vi "PSTR Controller.vi"(11 "Expt State (in)":T6) -> (3 "Expt State":T6)   [LabVIEW 2020]
uses:
  CFTS Main Panel SubVIs/CFTS-Experiment State.ctl
  epl-vi-lib/Utility VIs/Type Defs/Left-Right ring.ctl
  <vilib>/printing/EasyPrintingControls.llb/layout_options.ctl
  <vilib>/printing/EasyPrintingControls.llb/orientation.ctl
  <vilib>/printing/EasyPrintingControls.llb/panel_scaling_for_page.ctl
  <vilib>/printing/EasyPrintingControls.llb/margins.ctl
  <vilib>/printing/EasyPrintingControls.llb/margin_values.ctl
  <vilib>/printing/EasyPrintingControls.llb/measurement_system.ctl
  <vilib>/printing/EasyPrintingControls.llb/printer_options.ctl
  <vilib>/printing/EasyPrintingControls.llb/printing_method.ctl
  <vilib>/printing/EasyPrintingControls.llb/color_or_monochrome.ctl
  <vilib>/printing/EasyPrintingControls.llb/page_header_options.ctl
  <vilib>/printing/EasyPrintingControls.llb/page_headers.ctl
  <vilib>/printing/EasyPrintingControls.llb/page_header_content_options.ctl
  epl-vi-lib/Utility VIs/Buttons/KCheckmarkBoolean 2.ctl
  Typedefs/PSTR-Parameters.ctl
  Typedefs/PSTR-Stimulus Params.ctl
  Typedefs/PSTR-FreqSeq Params.ctl
  Typedefs/PSTR-LevelSeq Params.ctl
  Typedefs/PSTR-SeqParams.ctl
  Typedefs/PSTR-Response Params.ctl
  Typedefs/PSTR-Hidden Params.ctl
  Typedefs/PSTR-Window Shape.ctl
  Typedefs/PSTR-Data.ctl
  Typedefs/PSTR-Model Fit.ctl
  Typedefs/PSTR-Fit Parameters.ctl
  <vilib>/printing/EasyPrintingControls.llb/contents.ctl
  Typedefs/PSTR-Measurement State.ctl
  <vilib>/printing/EasyPrinting.llb/Easy Print VI Panel or Documentation (refnum).vi
  <vilib>/Utility/NIReport.llb/NI_ReportGenerationCore.lvlib
panel:
  in  "LevelSeq":T1={"Min (dB)"=0.0, "Max (dB)"=80.0, "Step (dB)"=20.0}
  in  "FreqSeq":T2={"Min (kHz)"=4.0, "Max (kHz)"=64.0, "Step (oct)"=0.5}
  in  "Seq":T3={"Order"=enum."Sequential", "Averages"=20}
  in  "Response":cluster{"Grass gain":dbl, "Window (ms)":dbl}={"Grass gain"=10000.0, "Window (ms)"=10000.0}
  in  "Stim":T5={"Ear"=enum."Right", "BW (oct)"=0.25, "Seed"=37, "Ramp (ms)"=5.0, "On time (ms)"=300.0, "Off time (ms)"=300.0, "Delay (ms)"=5.0}
  out "User":string
  out "Run #":u16
  out "ID #":u16
  out "Path":path
  out "Result":T7
  in  "Tab":enum32{"Recording", "Gain", "PSTR"}(tab)
  out "reject":bool
  out "Status":string
  out "Waveform":cluster{dbl, "dx":dbl, "Y":dbl[]}[](graph)
  out "Spectrum":cluster{dbl, "dx":dbl, "Y":dbl[]}[](graph)
  in  "RejThr":dbl=30.0 caption="Rej Thresh µV"
  in  "Override":bool
  in  "iFreq":u16(ring) items=["0.75 kHz"]
  out "Gain":cluster{"Array":dbl[], "Array":dbl[]}[](graph)
  in  "Legend":i32(listbox)
  out "vsFreq":cluster{"Array":dbl[], "Array":dbl[]}[](graph)
  in  "Show fits":T8
  in  "iFreq 2":u16(ring) items=["0.75 kHz"]
  in  "Legend 2":i32(listbox)
  out "PSTH":cluster{"Array":dbl[], "Array":dbl[]}[](graph)
  in  "Separation (uV)":dbl
  out "FitSummary":cluster{"Array":dbl[], "Array":dbl[]}[](graph)
  in  "Start":bool
  in  "Stop":bool
  out "Progress":cluster{"freq":i32, "level":i32} {"level" scale=0.0..2.0; "freq" scale=0.0..1.0}
  in  "layout options":T9={"orientation (unchanged)"=0, "panel scaling for page (unchanged)"=0, "margins"={"override VI margins (false)"=FALSE, "margins (1.00)"={"top"=1.0, "left"=1.0, "right"=1.0, "bottom"=1.0}, "measurement system (default)"=0}, "printer options"={"destination printer name (current)"="", "printing method (unchanged)"=0, "color or monochrome (unchanged)"=0}, "page header options"={"page headers (unchanged)"=0, "page header content options"={"Include VI Name"=TRUE, "Include VI Path"=TRUE, "Include Last Modification Date"=TRUE, "Include Date Printed"=TRUE, "Include Page Number"=TRUE, "Include VI Icon"=TRUE}}} {"page header options"."page headers (unchanged)" items=["Unchanged", "Include page headers", "Do not include page headers"]; "printer options"."color or monochrome (unchanged)" items=["Unchanged", "Color/grayscale", "Monochrome"]; "printer options"."printing method (unchanged)" items=["Unchanged", "Standard", "PostScript", "Bitmap"]; "panel scaling for page (unchanged)" items=["Unchanged", "No Scaling", "Scale front panel to fit"]; "orientation (unchanged)" items=["Unchanged", "portrait", "landscape"]; "margins"."measurement system (default)" items=["Default", "US", "Metric"]; "margins"."margins (1.00)"."right" format="%.2f"; "margins"."margins (1.00)"."bottom" format="%.2f"; "margins"."margins (1.00)"."top" format="%.2f"; "margins"."margins (1.00)"."left" format="%.2f"}
  in  "RETURN":bool
  # "Stimulus"
  # "Frequency"
  # "Level"
  # "Sequence"
  # "Response"
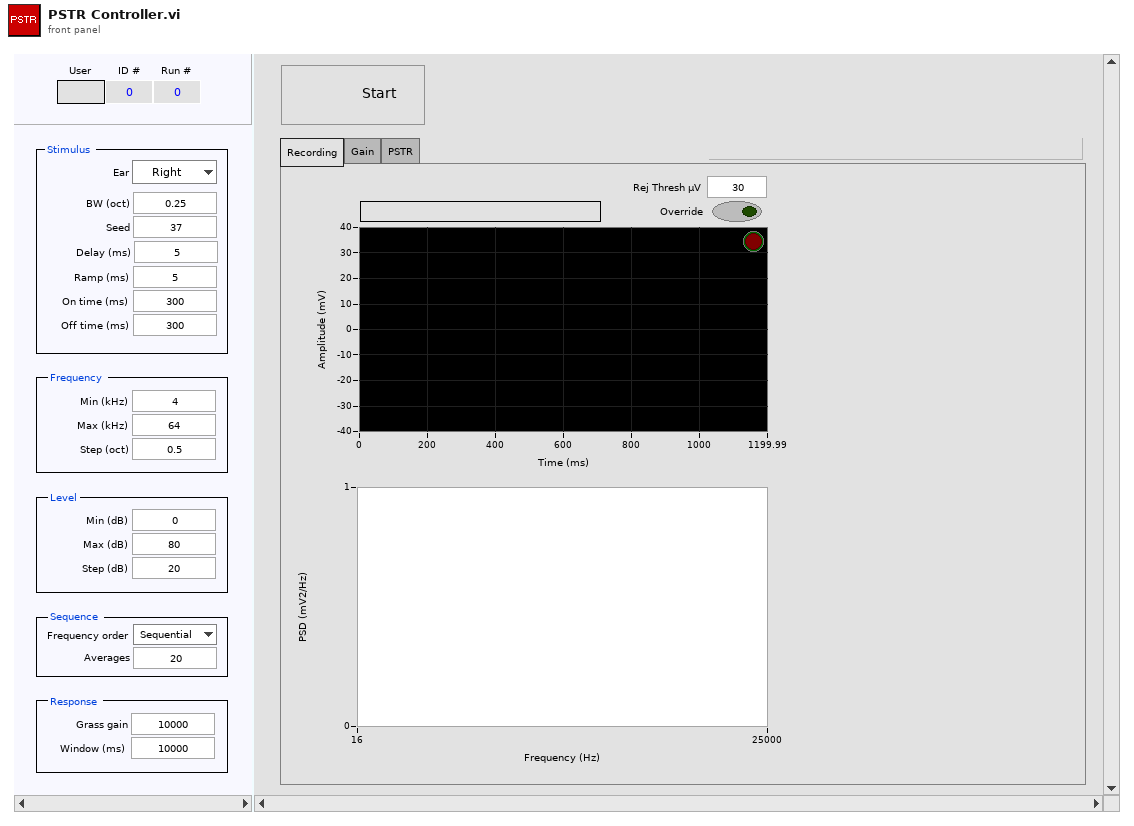
[diagram p1: front panel]
types:
  T1 = cluster{"Min (dB)":dbl, "Max (dB)":dbl, "Step (dB)":dbl}
  T2 = cluster{"Min (kHz)":dbl, "Max (kHz)":dbl, "Step (oct)":dbl}
  T3 = cluster{"Order":enum16{"Sequential", "Random"}, "Averages":i32}
  T4 = typedef "Left-Right ring.ctl" = enum16{"Right", "Left"}
  T5 = cluster{"Ear":T4, "BW (oct)":dbl, "Seed":i32, "Ramp (ms)":dbl, "On time (ms)":dbl, "Off time (ms)":dbl, "Delay (ms)":dbl}
  T6 = typedef "CFTS-Experiment State.ctl" = cluster{"Experimenter":string, "Number":u32, "Right":string, "Left":string, "Data Folder":path, "State File":path, "Version Info":string, "End Exposure Time":dbl, "Exposure Duration":string, "Run #":cluster{"CAP":i16, "ABR":i16, "DP":i16, "VsEP":i16, "MeasSeq":i16, "SubSeq":i16, "SFOAE":i16}}
  T7 = cluster{"iLevel":i32, "done":bool, "abort":bool, "PSD":dbl[][], "error":errorcluster, "spont":bool, "PSTH":dbl[]}
  T8 = typedef "KCheckmarkBoolean 2.ctl" = bool
  T9 = typedef "NI_ReportGenerationCore.lvlib/layout_options.ctl" = cluster{"orientation (unchanged)":T10, "panel scaling for page (unchanged)":T11, "margins":T12, "printer options":T15, "page header options":T18}
  T10 = typedef "NI_ReportGenerationCore.lvlib/orientation.ctl" = u16
  T11 = typedef "NI_ReportGenerationCore.lvlib/panel_scaling_for_page.ctl" = u16
  T12 = typedef "NI_ReportGenerationCore.lvlib/margins.ctl" = cluster{"override VI margins (false)":bool, "margins (1.00)":T13, "measurement system (default)":T14}
  T13 = typedef "NI_ReportGenerationCore.lvlib/margin_values.ctl" = cluster{"top":dbl, "left":dbl, "right":dbl, "bottom":dbl}
  T14 = typedef "NI_ReportGenerationCore.lvlib/measurement_system.ctl" = u16
  T15 = typedef "NI_ReportGenerationCore.lvlib/printer_options.ctl" = cluster{"destination printer name (current)":string, "printing method (unchanged)":T16, "color or monochrome (unchanged)":T17}
  T16 = typedef "NI_ReportGenerationCore.lvlib/printing_method.ctl" = u16
  T17 = typedef "NI_ReportGenerationCore.lvlib/color_or_monochrome.ctl" = u16
  T18 = typedef "NI_ReportGenerationCore.lvlib/page_header_options.ctl" = cluster{"page headers (unchanged)":T19, "page header content options":T20}
  T19 = typedef "NI_ReportGenerationCore.lvlib/page_headers.ctl" = u16
  T20 = typedef "NI_ReportGenerationCore.lvlib/page_header_content_options.ctl" = cluster{"Include VI Name":bool, "Include VI Path":bool, "Include Last Modification Date":bool, "Include Date Printed":bool, "Include Page Number":bool, "Include VI Icon":bool}
  T21 = typedef "PSTR-Data.ctl" = cluster{"Freq":dbl[], "Level":dbl[], "order":i32[], "PSD":dbl[][][][], "Gain":dbl[][][], "Index":dbl[][], "iFreq":i32, "df":dbl, "User":string, "ID":i32, "Run":i32, "iLevel":i32, "finished":bool, "resumed":bool, "Spont":dbl[][], "PSTR":dbl[][][], "dt":dbl, "delay":dbl, "durat":dbl, "Fits":T22[][], "Amplitude":dbl[][]}
  T22 = typedef "PSTR-Model Fit.ctl" = cluster{"Parameters":T23, "t":dbl[], "y":dbl[], "R2":dbl}
  T23 = typedef "PSTR-Fit Parameters.ctl" = cluster{"Ar":dbl, "Tr":dbl, "Ast":dbl, "Tst":dbl, "Ass":dbl}
  T24 = typedef "PSTR-Parameters.ctl" = cluster{"Stimulus":T25, "FreqSeq":T26, "LevelSeq":T27, "Seq":T28, "Response":T29, "Hidden":T30, "RejThr":dbl}
  T25 = typedef "PSTR-Stimulus Params.ctl" = cluster{"Ear":T4, "BW (oct)":dbl, "Seed":i32, "Ramp (ms)":dbl, "On time (ms)":dbl, "Off time (ms)":dbl, "Delay (ms)":dbl}
  T26 = typedef "PSTR-FreqSeq Params.ctl" = cluster{"Min (kHz)":dbl, "Max (kHz)":dbl, "Step (oct)":dbl}
  T27 = typedef "PSTR-LevelSeq Params.ctl" = cluster{"Min (dB)":dbl, "Max (dB)":dbl, "Step (dB)":dbl}
  T28 = typedef "PSTR-SeqParams.ctl" = cluster{"Order":enum16{"Sequential", "Random"}, "Averages":i32}
  T29 = typedef "PSTR-Response Params.ctl" = cluster{"Grass gain":dbl, "Window (ms)":dbl}
  T30 = typedef "PSTR-Hidden Params.ctl" = cluster{"Sample rate (Hz)":dbl, "Nfft":i32, "save raw":bool, "sep":dbl, "Window":T31}
  T31 = typedef "PSTR-Window Shape.ctl" = enum16{"NONE", "Hamming"}
  T32 = enum8{"Enabled", "Disabled", "Disabled and Grayed Out"}
  T33 = typedef "NI_ReportGenerationCore.lvlib/contents.ctl" = u16
  T34 = cluster{"PSTR Params":T24, "Freq":dbl, i32, "Run":i32}
  T35 = cluster{"PSTR Params":T24, "Freq":dbl, "iLevel":i32, "Run":i32}
  T36 = typedef "PSTR-Measurement State.ctl" = enum16{"Init", "Next", "Measure", "End"}
  T37 = enum16{"open", "replace", "create", "open or create", "replace or create", "replace or create with confirmation"}
  T38 = typedef "PSTR-Runtime Data.ctl" = cluster{"Fs":dbl, "AOpts":i32, "stimChan":T39, "len":i32, "offset1":i32, "iLevel":i32, "AOChan":i32[], "Level":dbl[], "nacc":i32, "nrej":i32, "nacq":i32, "abort":bool, "offset2":i32, "gain":dbl, "Nfft":i32, "Neural":dbl[], "Micro":dbl[], "raw":refnum<file>, "spont":bool, "PSTR":dbl[], "trialLen":i32, "gate":dbl[], "window":u16, "BP":cluster{"reverse":dbl[], "forward":dbl[]}, "Smooth":cluster{"reverse":dbl[], "forward":dbl[]}}
  T39 = typedef "Stimulus Channel (Full).xctl/Full Stimulus Channel Data.ctl" = cluster{"Waveform":T40, "Filter":T57, "Burst":T59, "Level":T60, "Name":string, "Advanced":T62, "SAM":T63}
  T40 = typedef "Waveform XCtl.xctl/Waveform Data.ctl" = cluster{"Type":T41, "Tone":T42, "Pulse Train":T43, "Noise":T46, "File":T47, "FMSweep":T48, "Chirp Train":T49, "Complex Tone":cluster{"Params":T51, "Data":T53}, "Moving Ripple":T54}
  T41 = typedef "Waveform Enum.ctl" = enum16{"OFF", "Tone", "Noise", "Pulse Train", "File", "FM Sweep", "Chirp Train", "Complex Tone", "FM Tone", "Moving Ripple"}
  T42 = typedef "Tone Params.ctl" = cluster{"Frequency (kHz)":dbl, "Last Freq":dbl, "Last Phase":dbl}
  T43 = typedef "Pulse Train Params.ctl" = cluster{"Pulse width (us)":dbl, "Pulse rate (Hz)":dbl, "Gap (ms)":dbl, "Polarity":T44, "PT State":T45, "Asynch":bool}
  T44 = typedef "Pulse Polarity.ctl" = enum16{"POS", "NEG", "POS-NEG", "NEG-POS"}
  T45 = typedef "PT-Continuous State.ctl" = cluster{"Template":dbl[], "Nperiod":i32, "Index":i32, "Pulse Rate (Hz)":dbl, "Phase (cycles)":dbl, "Noff":i32}
  T46 = typedef "Noise Params.ctl" = cluster{"InvFilt":bool, "Noise":dbl[], "CurPt":i32, "Aweight":bool, "Seed":i32, "afile":path}
  T47 = typedef "StimFile-Params.ctl" = cluster{"Filename":path, "Signal":dbl[], "Channel":i32, "stream":bool, "offset":i32, "nreps":i32, "loops":i32, "Randomize":bool, "order":i32[], "Seed":i32, "Tokens":i32}
  T48 = typedef "FM Sweep Params.ctl" = cluster{"Rate (oct/s)":dbl, "Fmin (Hz)":dbl, "Fmax (Hz)":dbl, "Ramp (ms)":dbl, "Linear":bool}
  T49 = typedef "Chirp Train.ctl" = cluster{"Params":T50, "Data":cluster{"WF":dbl[]}}
  T50 = typedef "Chirp Train Params.ctl" = cluster{"Fmin (kHz)":dbl, "Fmax (kHz)":dbl, "Compensate":bool, "Duration (ms)":dbl}
  T51 = typedef "CT-Params.ctl" = cluster{"F0 (Hz)":dbl, "Band":cluster{"Flow (Hz)":dbl, "Fhigh (Hz)":dbl}, "Phase":T52, "Min F0 (Hz)":dbl, "Max F0 (Hz)":dbl, "ContinRandPhase":bool, "Max peak factor":dbl, "Max mod depth":dbl, "MinHarmNum":i32, "MaxHarmNum":i32, "Level Mode":enum16{"per component", "overall rms"}, "% jitter":dbl}
  T52 = typedef "CT-Phase Enum.ctl" = enum16{"Cosine", "Random", "Alternating"}
  T53 = typedef "CT-Runtime Data.ctl" = cluster{"Ncomp":i32, "MinHarm":i32, "Phase":dbl[], "Amplitude":dbl[], "Npts/frame":i32, "Last F0":dbl, "Fmin":dbl, "Fmax":dbl, "Lslope":dbl, "randphase":bool, "overall rms":bool, "fmult":dbl[], "jittered":bool}
  T54 = typedef "Moving Ripple.ctl" = cluster{"Params":T55, "Data":T56}
  T55 = typedef "Moving Ripple.Params.ctl" = cluster{"Fmin":dbl, "Fmax":dbl, "Density":dbl, "Velocity":dbl, "Depth":dbl, "Phase":dbl, "Comp/oct":i32}
  T56 = typedef "Moving Ripple.Data.ctl" = cluster{"Freq":dbl[], "A":dbl[], "phase":dbl[], "Phase":dbl}
  T57 = typedef "Advanced Filter XCtl.xctl/Filter Data.ctl" = cluster{"Type":enum16{"Lowpass", "Highpass", "Bandpass", "Bandstop", "OFF"}, "CF (kHz)":dbl, "BW (kHz)":dbl, "Cascade":bool, "Quadrature":bool, "Scale Factor":dbl, "Stages":cluster{"IIR Filter":cluster{"filter structure":enum32{"IIR 2nd Order", "IIR 4th Order"}, "Reverse Coefficients":dbl[], "Forward Coefficients":dbl[]}, "State":dbl[]}[], "Class":enum16{"Elliptic", "Butterworth"}, "Order":i32, "BWUnits":T58}
  T58 = typedef "Filter-Bandwidth Units.ctl" = enum16{"Linear", "Octaves", "Min-Max"}
  T59 = typedef "Burst Control.xctl/Burst Data.ctl" = cluster{"Active":bool, "Delay (ms)":dbl, "Duration (ms)":dbl, "Ramp (ms)":dbl, "Rate (Hz)":dbl, "Trepeat (ms)":dbl, "Repeat":bool}
  T60 = typedef "Level XCtl.xctl/Level Data.ctl" = cluster{"Level":dbl, "Units":T61, "Max":dbl, "Multiplier":dbl, "Cal File":path, "Cal":cluster{"Freq (Hz)":dbl[], "Mag (dB SPL)":dbl[], "Phase (deg)":dbl[]}}
  T61 = typedef "Level Units.ctl" = enum16{"dB atten", "dB SPL", "dB re 1 Vrms", "dB V/Hz½", "mW", "dB HL", "Volts", "dB mW"}
  T62 = typedef "Advanced Stimulus Options.xctl/Advanced Stimulus Options.ctl" = cluster{"Rep Mask":string, "AltPol":bool, "Var":string, "Expr":string, "Persist":bool}
  T63 = typedef "SAM Params.ctl" = cluster{"Active":bool, "Frequency (Hz)":dbl, "Depth":dbl, "Init Phase (cycles)":dbl, "phase (degrees)":dbl, "Asynch":bool}
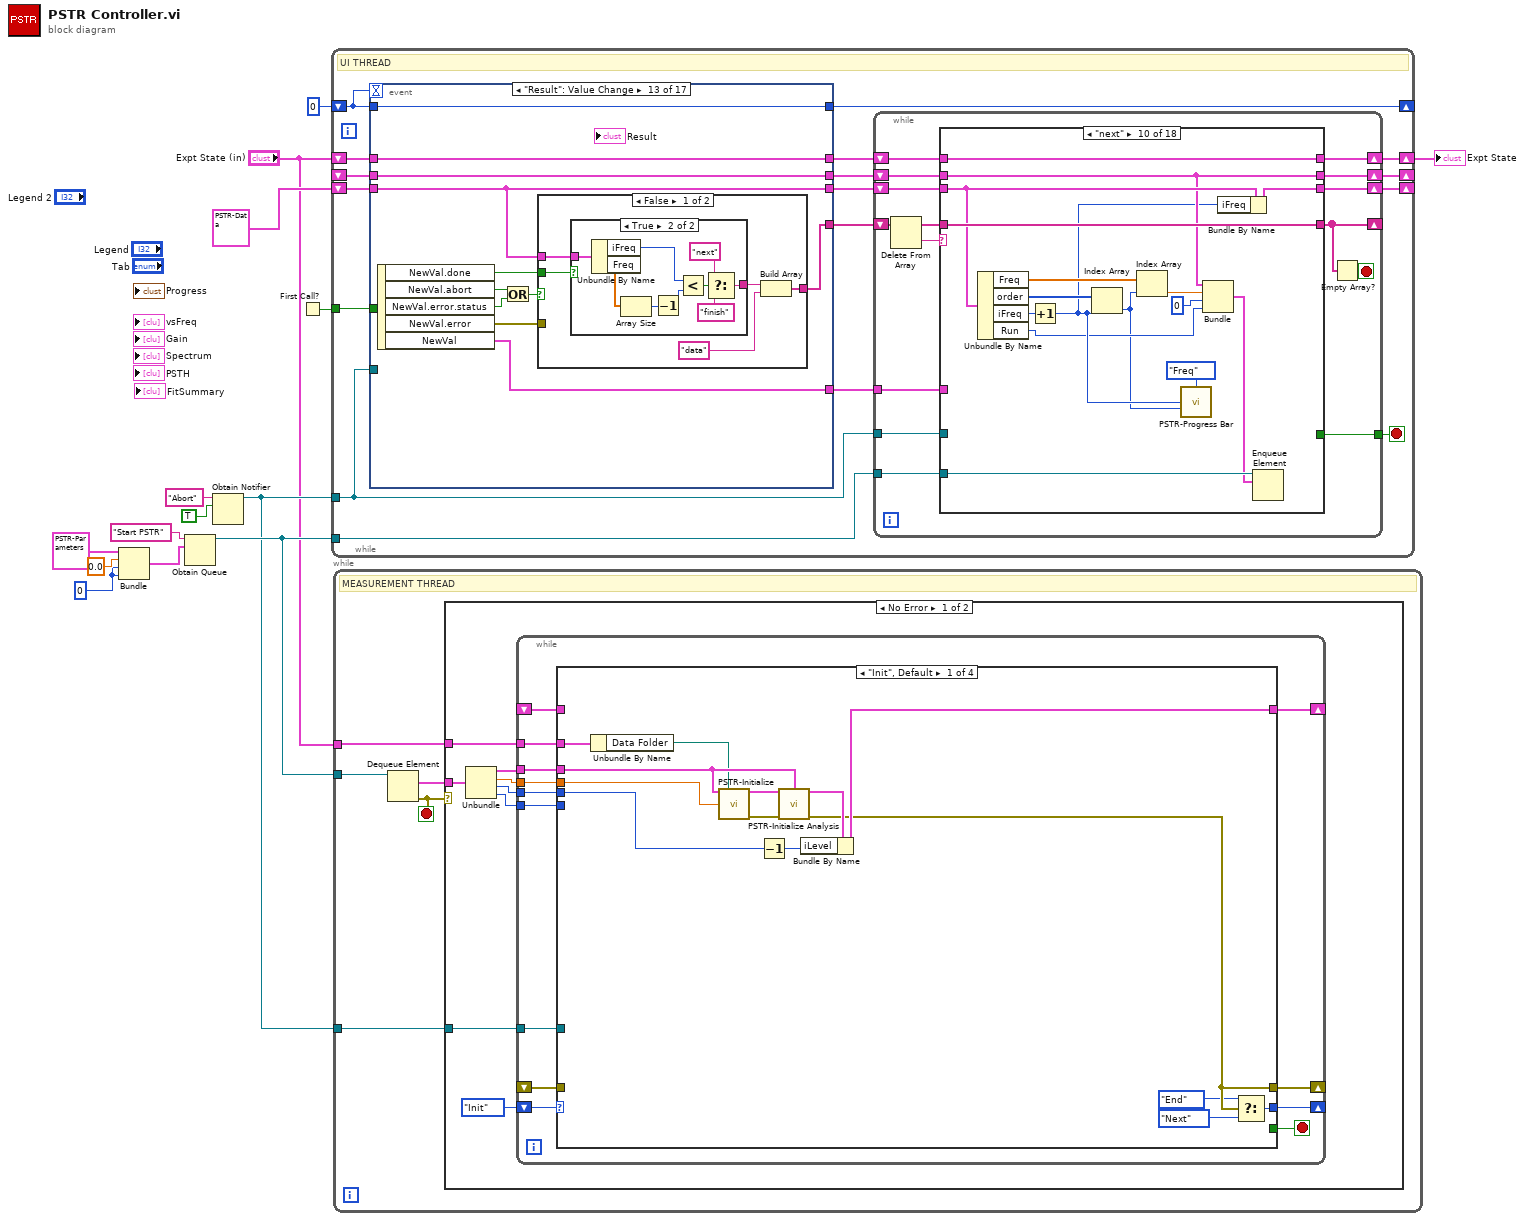
[diagram p0: block diagram]
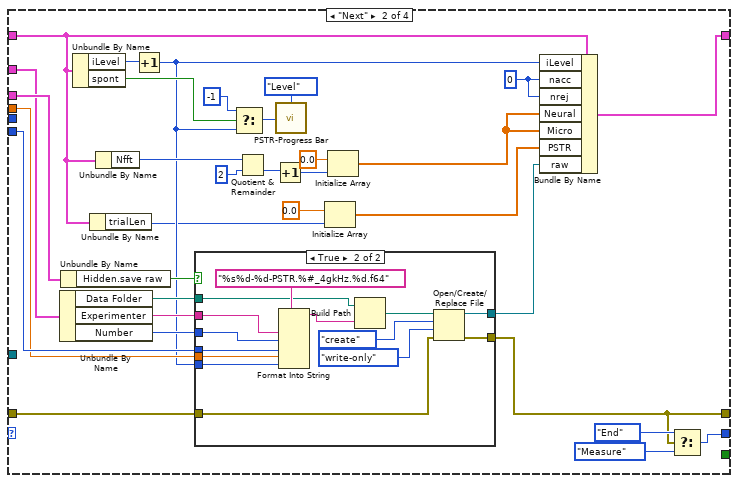
[diagram p2: hidden frame]
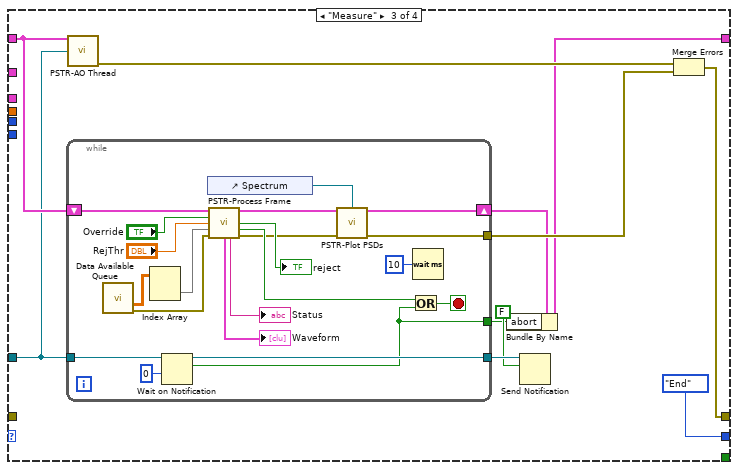
[diagram p4: hidden frame]
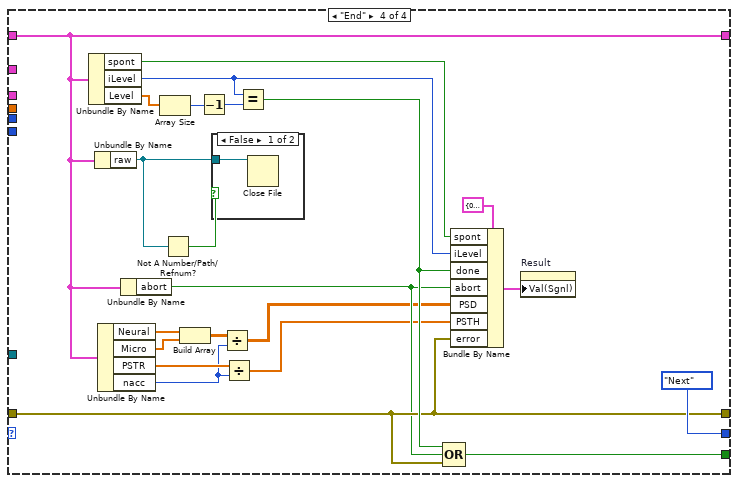
[diagram p5: hidden frame]
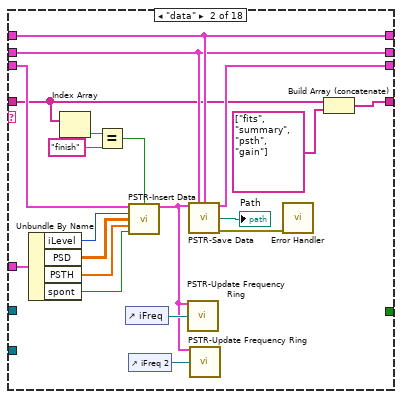
[diagram p9: hidden frame]
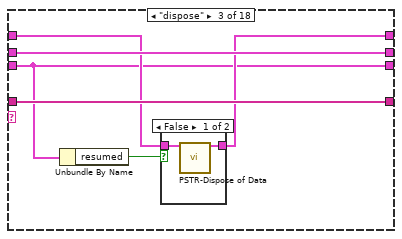
[diagram p10: hidden frame]
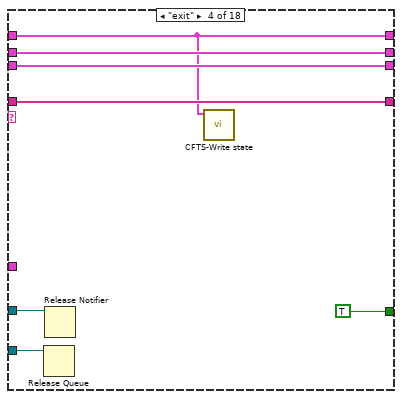
[diagram p12: hidden frame]
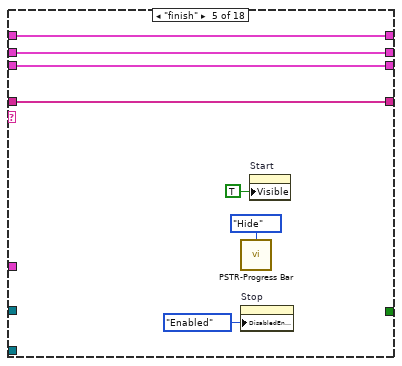
[diagram p13: hidden frame]
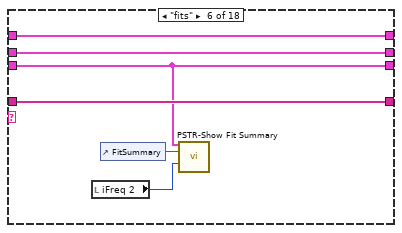
[diagram p14: hidden frame]
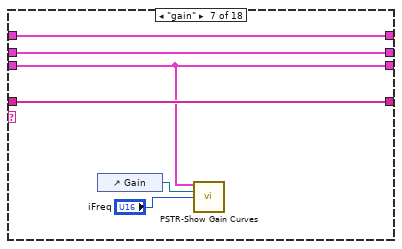
[diagram p15: hidden frame]
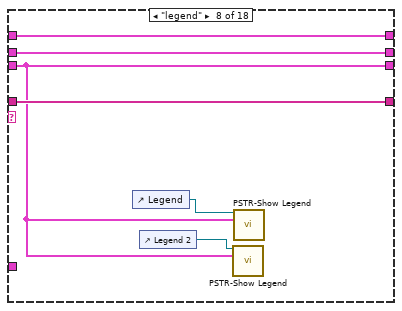
[diagram p16: hidden frame]
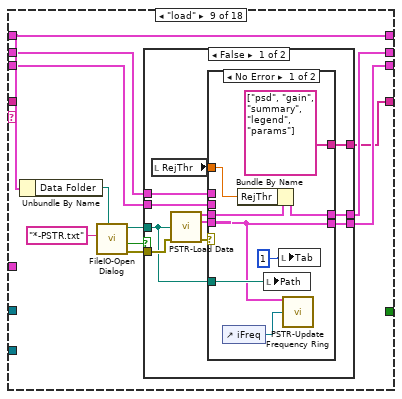
[diagram p17: hidden frame]
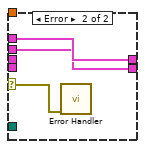
[diagram p18: hidden frame]
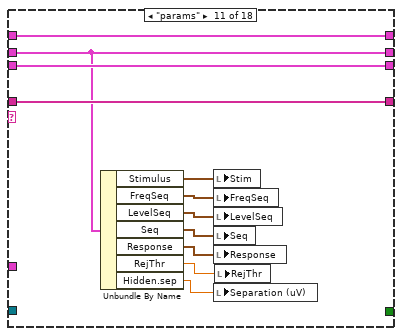
[diagram p20: hidden frame]
diagram:
  w2 = 0
  n1 = Bundle("PSTR Params"=T24 {"Stimulus"={"Ear"=enum."Right", "BW (oct)"=673.0, "Seed"=6, "Ramp (ms)"=10000.0, "On time (ms)"=10000.0, "Off time (ms)"=10000.0, "Delay (ms)"=10000.0}, "FreqSeq"={"Min (kHz)"=10000.0, "Max (kHz)"=10000.0, "Step (oct)"=10000.0}, "LevelSeq"={"Min (dB)"=10000.0, "Max (dB)"=10000.0, "Step (dB)"=10000.0}, "Seq"={"Order"=enum."Sequential", "Averages"=6}, "Response"={"Grass gain"=10000.0, "Window (ms)"=0.0}, "Hidden"={"Sample rate (Hz)"=20000.0, "Nfft"=0, "save raw"=FALSE, "sep"=0.0, "Window"=enum."NONE"}, "RejThr"=0.0}, 0.0, w2, w2) -> (w8:cluster{"PSTR Params":T24, dbl, i32, i32})  [unwired: 1 in]
  n2 = Obtain Queue(name (unnamed)="Start PSTR", element data type=w8) -> (queue out=w14:refnum<queue>)  [unwired: 3 in, 2 out]
  n3 = Obtain Notifier(name (unnamed)="Abort", notification data type=TRUE) -> (notifier out=w3:refnum<notifier>)  [unwired: 2 in, 2 out]
  n4 = First Call?() -> (First Call?: T/F=w11:bool)
  n5 = while {
    tunnel: w14 -> [w15]
    shift-right: [w31] -> _
    shift-left: 0 -> [w27]
    tunnel: w11 -> [w30]
    shift-right: [w22] -> w10
    shift-left: "Expt State (in)" -> [w29]
    shift-right: [w24] -> _
    shift-left: _ -> [w28]
    shift-right: [w18] -> _
    shift-left: T21 {"Freq"=[], "Level"=[], "order"=[], "PSD"=[], "Gain"=[], "Index"=[], "iFreq"=0, "df"=0.0, "User"="", "ID"=0, "Run"=0, "iLevel"=0, "finished"=FALSE, "resumed"=FALSE, "Spont"=[], "PSTR"=[], "dt"=0.0, "delay"=0.0, "durat"=0.0, "Fits"=[], "Amplitude"=[]} ("Data") -> [w20]
    tunnel: w3 -> [w16]
    stop <- w21 stop-if-true
    # "UI THREAD"
    n6 = event shown="[12] \"Result\": Value Change" {
      selector: _ -> [_ _ _ _ _ _ _ _ _ _ _ _ _ _ _ _ _]
      dyn-events: _ -> [_ _ _ _ _ _ _ _ _ _ _ _ _ _ _ _ _]
      timeout: w27 -> [_ _ _ w344 _ _ _ _ _ _ _ _ _ _ _ _ _]
      tunnel: [-1 w303 w307 w344 w348 w352 w358 w364 w370 w376 w387 w395 w407 w428 w433 w440 w445] -> w31
      tunnel: w30 -> [w280 _ _ _ _ _ _ _ _ _ _ _ _ _ _ _ _]
      tunnel: w29 -> [w283 w298 w306 w340 w347 w351 w357 w363 w369 w375 w386 w394 w406 w427 w432 w439 w444]
      tunnel: [w283 w298 w306 w340 w347 w351 w357 w363 w369 w375 w386 w394 w406 w427 w432 w439 w444] -> w23
      tunnel: w28 -> [w282 w302 w309 w342 w349 w355 w361 w367 w373 w379 w388 w396 w405 w426 w431 w438 w443]
      tunnel: [w282 w302 w308 w342 w349 w354 w360 w366 w372 w378 w388 w396 w405 w426 w431 w435 w443] -> w25
      tunnel: w27 -> [_ w303 w307 _ w348 w352 w358 w364 w370 w376 w387 w395 w407 w428 w433 w440 w445]
      tunnel: [w278 _ w305 string[] ["exit"] ("f") string[] ["exit"] ("f") _ _ _ _ _ string[] ["start"] ("f") _ w397 string[] ["gain"] ("f") string[] ["fits", "psth"] ("f") string[] ["psth"] ("f") string[] ["psth"] ("f")] -> w26
      tunnel: w20 -> [w277 w297 w304 w339 w345 w350 w356 w362 w368 w374 w384 w393 w399 w425 w430 w437 w442]
      tunnel: [w277 w297 w304 w339 w345 w350 w356 w362 w368 w374 w384 w393 w399 w425 w430 w437 w442] -> w19
      tunnel: [_ _ _ _ _ _ _ _ _ _ _ _ w403 _ _ _ _] -> w17
      tunnel: w16 -> [_ _ _ _ _ _ _ _ _ _ w381 w392 _ _ _ _ _]
      event Timeout {
        n7 = event-data() -> ()  [unwired: 1 in, 1 out]
        n8 = control-ref of="Progress"() -> (w276:refnum<vi>)
        n9 = Unbundle By Name(w283) -> ("Experimenter"=→"User":string, "Number"=→"ID #":u32, "Run #.CAP"=→"Run #":i16)
        n10 = call "PSTR-Progress Bar.vi"("Action"=enum16{"Init", "Seq", "Freq", "Level", "Hide"}."Init", "Progress"=w276) -> ()  [unwired: 13 in, 1 out]
        n11 = property on="Start" class="Bool"("Visible"=TRUE) -> ()  [unwired: 2 in, 2 out]
        n12 = property on="Stop" class="Bool"("DisabledEnum"=T32."Enabled" ("Disabled")) -> ()  [unwired: 2 in, 2 out]
        n13 = local write "Path"(path "" ("Path")) -> ()
        n14 = Select(t=string[] ["restore"], s=w280, f=string[] []) -> (s? t:f=w278:string[])
      }
      event Menu Activation? {
        n15 = event-data() -> ("MenuRef"=w300:refnum<k9>)  [unwired: 1 in]
        n16 = Unbundle By Name(w297) -> ("User"=w295:string, "ID"=w292:i32, "finished"=w290:bool)
        n17 = Unbundle By Name(w298) -> ("Experimenter"=w296:string, "Number"=w293:u32)
        n18 = Equal?(x=w296, y=w295) -> (x = y?=w294:bool)
        n19 = Equal?(x=w293, y=w292) -> (x = y?=w291:bool)
        n20 = Compound Arithmetic op=AND(w294, w291, invert w290) -> (w289:bool)
        n21 = Set Menu Item Info(7:"mmFileResume" ("item tag"), 9:w289, 11:w300) -> ()  [unwired: 4 in, 2 out]
        n22 = event-data("Discard?"=FALSE) -> ()  [unwired: 1 in, 1 out]
      }
      event Menu Selection (User) {
        n23 = event-data() -> ("ItemTag"=w311:string)  [unwired: 1 in]
        n24 = case shown="\"mmOptions\"" w311 {
          tunnel: [_ _ w317 _ _ w329 _ _] -> w310
          tunnel: w309 -> [w312 w314 w319 w325 w327 w328 w334 w338]
          tunnel: [w312 w314 w319 w325 w327 w328 w334 w336] -> w308
          tunnel: [_ string[] ["restore"] _ string[] ["load"] string[] ["resume"] _ string[] ["exit"] _] -> w305
          frame "", Default {
          }
          frame "mmFileRestore" {
          }
          frame "mmFileSave" {
            n25 = local read "RejThr"() -> (w315:dbl)
            n26 = Bundle By Name(cluster=w319, "RejThr"=w315) -> (w316:T24)
            n27 = call "Default Config File Path.vi"() -> ("Default config file name"=w321:path)
            n28 = call "Write Anything.vi"("Section Name (Name of \"Anything\")"="PSTR" ("Section Name (Name of \"Anything\")"), "Anything"=w316, "Path (dialog)"=w321) -> ("Error Out"=w318:errorcluster)  [unwired: 7 in, 1 out]
            n29 = case shown="No Error" w318 {
              selector: w318 -> [_ w323]
              tunnel: [_ w323] -> w317
              frame No Error {
                n30 = One Button Dialog(message="Defaults saved.") -> ()  [unwired: 1 in, 1 out]
              }
              frame Error {
              }
            }
          }
          frame "mmFileLoad" {
          }
          frame "mmFileResume" {
          }
          frame "mmFilePrint" {
            w331 = T33 1 items=["Complete front panel", "Visible portion of front panel", "Icon, description, panel and diagram", "Documentation: Using the panel", "Documentation: Using as a subVI", "Documentation: Complete", "Documentation: Custom"] ("contents (complete front panel)")
            n31 = control-ref of="This VI"() -> (w330:refnum<vi>)
            n32 = call-poly <vilib>:"Easy Print VI Panel or Documentation.vi"("layout options"="layout options", "contents (complete front panel)"=w331, "VI reference"=w330) -> ("error out"=w329:errorcluster)  [unwired: 7 in, 1 out]
          }
          frame "mmFileExit" {
          }
          frame "mmOptions" {
            n33 = Unbundle By Name(w338) -> ("Hidden"=w337:T30)
            n34 = call "PSTR-Options Dialog.vi"("Cluster In"=w337) -> ("Cluster out"=w335:T30)  [unwired: 13 in, 1 out]
            n35 = Bundle By Name(cluster=w338, "Hidden"=w335) -> (w336:T24)
          }
        }
        n36 = call "Error Handler.vi"("error in (no error)"=w310) -> ()  [unwired: 13 in, 2 out]
      }
      event Panel Close? {
        n37 = event-data() -> ()  [unwired: 1 in, 1 out]
        n38 = event-data("Discard?"=TRUE) -> ()  [unwired: 1 in, 1 out]
      }
      event "RETURN": Value Change {
        n39 = event-data() -> ()  [unwired: 1 in, 1 out]
      }
      event "Stim": Value Change {
        n40 = event-data() -> ()  [unwired: 1 in, 1 out]
        n41 = Bundle By Name(cluster=w355, "Stimulus"="Stim") -> (w354:T24)
      }
      event "FreqSeq": Value Change {
        n42 = event-data() -> ()  [unwired: 1 in, 1 out]
        n43 = Bundle By Name(cluster=w361, "FreqSeq"="FreqSeq") -> (w360:T24)
      }
      event "LevelSeq": Value Change {
        n44 = event-data() -> ()  [unwired: 1 in, 1 out]
        n45 = Bundle By Name(cluster=w367, "LevelSeq"="LevelSeq") -> (w366:T24)
      }
      event "Seq": Value Change {
        n46 = event-data() -> ()  [unwired: 1 in, 1 out]
        n47 = Bundle By Name(cluster=w373, "Seq"="Seq") -> (w372:T24)
      }
      event "Response": Value Change {
        n48 = event-data() -> ()  [unwired: 1 in, 1 out]
        n49 = Bundle By Name(cluster=w379, "Response"="Response") -> (w378:T24)
      }
      event "Start": Value Change {
        w382 = cluster{dbl, "dx":dbl, "Y":dbl[]}[] [] ("Waveform")
        n50 = event-data() -> ()  [unwired: 1 in, 1 out]
        n51 = Cancel Notification(0:w381) -> ()  [unwired: 1 in, 3 out]
        n52 = property on="Start" class="Bool"("Visible"=FALSE) -> ()  [unwired: 2 in, 2 out]
        n53 = local write "Status"("" ("Status")) -> ()
        n54 = local write "Tab"(enum32{"Recording", "Gain", "PSTR"}."Recording" ("Tab")) -> ()
        n55 = local write "Waveform"(w382) -> ()
        n56 = local write "Spectrum"(w382) -> ()
      }
      event "Stop": Value Change {
        n57 = event-data() -> ()  [unwired: 1 in, 1 out]
        n58 = Send Notification(notification=TRUE, notifier=w392) -> ()  [unwired: 1 in, 2 out]
        n59 = property on="Stop" class="Bool"("DisabledEnum"=T32."Disabled and Grayed Out" ("Disabled")) -> ()  [unwired: 2 in, 2 out]
      }
      event "Result": Value Change {
        n60 = event-data() -> ("NewVal.done"=w404:bool, "NewVal.abort"=w401:bool, "NewVal.error.status"=w402:bool, "NewVal.error"=w398:errorcluster, "NewVal"=w403:T7)  [unwired: 1 in]
        n61 = Or(x=w401, y=w402) -> (x .or. y?=w400:bool)
        n62 = case shown="False" w400 {
          tunnel: w404 -> [w412 _]
          tunnel: [w408 string[] ["finish", "dispose"]] -> w397
          tunnel: w399 -> [w411 _]
          tunnel: w398 -> [_ w422]
          frame False {
            n63 = case shown="True" w412 {
              tunnel: w411 -> [_ w421]
              tunnel: [_ w415] -> w409
              frame False {
              }
              frame True {
                n64 = Unbundle By Name(w421) -> ("iFreq"=w420:i32, "Freq"=w414:dbl[])
                n65 = Array Size(array=w414) -> (size(s)=w419:i32)
                n66 = Decrement(x=w419) -> (x-1=w413:i32)
                n67 = Less?(x=w420, y=w413) -> (x < y?=w418:bool)
                n68 = Select(t="next" ("String"), s=w418, f="finish" ("String")) -> (s? t:f=w415:string)
              }
            }
            n69 = Build Array(w409, "data" ("String")) -> (w408:string[])
          }
          frame True {
            n70 = call "Error Handler.vi"("error in (no error)"=w422) -> ()  [unwired: 13 in, 2 out]
          }
        }
      }
      event "iFreq": Value Change {
        n71 = event-data() -> ()  [unwired: 1 in, 1 out]
      }
      event "iFreq 2": Value Change {
        n72 = event-data() -> ()  [unwired: 1 in, 1 out]
      }
      event "Separation (uV)": Value Change {
        n73 = event-data() -> ("NewVal"=w434:dbl)  [unwired: 1 in]
        n74 = Bundle By Name(cluster=w438, "Hidden.sep"=w434) -> (w435:T24)
      }
      event Value Change {
        n75 = event-data() -> ()  [unwired: 1 in, 1 out]
      }
    }
    n76 = while {
      shift-right: [w36] -> _
      shift-left: w26 -> [w46]
      shift-right: [w39] -> w24
      shift-left: w25 -> [w42]
      shift-right: [w40] -> w22
      shift-left: w23 -> [w41]
      tunnel: w15 -> [w38]
      tunnel: [w37] -> w21
      shift-right: [w34] -> w18
      shift-left: w19 -> [w35]
      tunnel: w17 -> [w33]
      tunnel: w16 -> [w32]
      stop <- w44 stop-if-true
      n77 = Delete From Array(array=w46) -> (deleted portion=w45:string, array with subset deleted=w43:string[])  [unwired: 2 in]
      n78 = case shown="\"next\"" w45 {
        tunnel: w43 -> [w48 w59 w75 w85 w91 w97 w103 w110 _ w162 w172 w176 w184 w198 _ w242 _ w270]
        tunnel: w42 -> [w49 w65 w76 w86 w92 w98 w104 w109 w114 w155 w164 w177 w185 _ w223 w239 w250 w271]
        tunnel: w41 -> [w50 w66 w74 w80 w93 w99 w105 w111 w121 w149 w173 w178 w186 w199 w229 w236 w244 w272]
        tunnel: [w50 w66 w73 w80 w93 w99 w105 w111 w121 w149 w173 w178 w186 w199 w229 w236 w243 w272] -> w40
        tunnel: [w49 w65 w76 w86 w92 w98 w104 w109 w113 w155 w164 w177 w185 w191 w223 w239 w250 w271] -> w39
        tunnel: [w48 w63 w75 w85 w91 w97 w103 w110 w112 w162 w172 w176 w184 w189 string[] ["legend"] w242 w245 w270] -> w36
        tunnel: w38 -> [_ _ _ w84 _ _ _ _ _ w157 _ _ _ _ w222 w240 _ _]
        tunnel: [_ _ _ TRUE _ _ _ _ _ _ _ _ _ _ _ _ _ _] -> w37
        tunnel: w35 -> [w47 w62 w72 w82 w90 w95 w100 w107 w117 w161 w165 w174 w182 w190 w209 w241 w248 w268]
        tunnel: [w47 w67 w72 w82 w90 w95 w100 w107 w116 w153 w165 w174 w182 w190 w215 w241 w247 w268] -> w34
        tunnel: w33 -> [_ w70 _ _ _ _ _ _ _ _ _ _ _ _ _ _ _ _]
        tunnel: w32 -> [_ _ _ w81 _ _ _ _ _ _ _ _ _ _ w213 _ _ _]
        frame "", Default {
        }
        frame "data" {
          n79 = Unbundle By Name(w70) -> ("iLevel"=w68:i32, "PSD"=w69:dbl[][], "PSTH"=w54:dbl[], "spont"=w55:bool)
          n80 = Index Array(array=w59) -> (element=w58:string)  [unwired: 1 in]
          n81 = Equal?(x=w58, y="finish") -> (x = y?=w56:bool)
          n82 = control-ref of="iFreq"() -> (w60:refnum<vi>)
          n83 = call "PSTR-Insert Data.vi"("Data in"=w62, "Finished"=w56, "iLevel"=w68, "PSD"=w69, "PSTR"=w54, "Spont"=w55) -> ("Data out"=w52:T21)  [unwired: 9 in]
          n84 = control-ref of="iFreq 2"() -> (w51:refnum<vi>)
          n85 = call "PSTR-Update Frequency Ring.vi"("Data"=w52, "Freq Ring"=w60) -> ()  [unwired: 14 in]
          n86 = call "PSTR-Save Data.vi"("Data in"=w52, "PSTR Params"=w65, "Expt State (in)"=w66) -> ("Data out"=w67:T21, "file path out"=→"Path":path, "Error Out"=w64:errorcluster)  [unwired: 10 in]
          n87 = call "PSTR-Update Frequency Ring.vi"("Data"=w52, "Freq Ring"=w51) -> ()  [unwired: 14 in]
          n88 = call "Error Handler.vi"("error in (no error)"=w64) -> ()  [unwired: 13 in, 2 out]
          n89 = Build Array (concatenate)(w59, string[] ["fits", "summary", "psth", "gain"]) -> (w63:string[])
        }
        frame "dispose" {
          n90 = Unbundle By Name(w72) -> ("resumed"=w71:bool)
          n91 = case shown="False" w71 {
            tunnel: w74 -> [w78 w79]
            tunnel: [w77 w79] -> w73
            frame False {
              n92 = call "PSTR-Dispose of Data.vi"("Expt State (in) in"=w78) -> ("Expt State (in) out"=w77:T6)  [unwired: 14 in]
            }
            frame True {
            }
          }
        }
        frame "exit" {
          n93 = Release Queue(queue=w84) -> ()  [unwired: 2 in, 3 out]
          n94 = Release Notifier(notifier=w81) -> ()  [unwired: 2 in, 3 out]
          n95 = call "CFTS-Write state.vi"("Experiment info"=w80) -> ()  [unwired: 10 in, 1 out]
        }
        frame "finish" {
          n96 = call "PSTR-Progress Bar.vi"("Action"=enum16{"Init", "Seq", "Freq", "Level", "Hide"}."Hide") -> ()  [unwired: 14 in, 1 out]
          n97 = property on="Stop" class="Bool"("DisabledEnum"=T32."Enabled" ("Disabled")) -> ()  [unwired: 2 in, 2 out]
          n98 = property on="Start" class="Bool"("Visible"=TRUE) -> ()  [unwired: 2 in, 2 out]
        }
        frame "fits" {
          n99 = local read "iFreq 2"() -> (w94:u16)
          n100 = control-ref of="FitSummary"() -> (w96:refnum<vi>)
          n101 = call "PSTR-Show Fit Summary.vi"("Data"=w95, "XYGraph"=w96, "Freq index"=w94) -> ()  [unwired: 13 in]
        }
        frame "gain" {
          n102 = control-ref of="Gain"() -> (w102:refnum<vi>)
          n103 = call "PSTR-Show Gain Curves.vi"("Data"=w100, "XYGraph"=w102, "Freq"="iFreq") -> ()  [unwired: 13 in]
        }
        frame "legend" {
          n104 = control-ref of="Legend"() -> (w108:refnum<vi>)
          n105 = control-ref of="Legend 2"() -> (w106:refnum<vi>)
          n106 = call "PSTR-Show Legend.vi"("ListBox in"=w106, "Data"=w107) -> ()  [unwired: 14 in]
          n107 = call "PSTR-Show Legend.vi"("ListBox in"=w108, "Data"=w107) -> ()  [unwired: 14 in]
        }
        frame "load" {
          n108 = Unbundle By Name(w121) -> ("Data Folder"=w120:path)
          n109 = call "FileIO-Open Dialog.vi"("Default Folder"=w120, "pattern (all files)"="*-PSTR.txt") -> ("error out"=w115:errorcluster, "cancelled"=w118:bool, "selected path"=w119:path)  [unwired: 7 in]
          n110 = case shown="False" w118 {
            tunnel: w119 -> [w124 _]
            tunnel: w117 -> [w129 w146]
            tunnel: [w130 w146] -> w116
            tunnel: w115 -> [w133 _]
            tunnel: w114 -> [w131 w145]
            tunnel: [w126 w145] -> w113
            tunnel: [w125 _] -> w112
            frame False {
              n111 = local read "RejThr"() -> (w123:dbl)
              n112 = call "PSTR-Load Data.vi"("selected path"=w124, "error in (no error)"=w133) -> ("Params"=w128:T24, "Data"=w127:T21, "error out"=w132:errorcluster)  [unwired: 10 in, 1 out]
              n113 = case shown="No Error" w132 {
                selector: w132 -> [_ w144]
                tunnel: w131 -> [_ w143]
                tunnel: [w135 w143] -> w126
                tunnel: [w137 w142] -> w130
                tunnel: w129 -> [_ w142]
                tunnel: w128 -> [w138 _]
                tunnel: w127 -> [w137 _]
                tunnel: [string[] ["psd", "gain", "summary", "legend", "params"] _] -> w125
                tunnel: w124 -> [w139 _]
                tunnel: w123 -> [w134 _]
                frame No Error {
                  n114 = control-ref of="iFreq"() -> (w136:refnum<vi>)
                  n115 = Bundle By Name(cluster=w138, "RejThr"=w134) -> (w135:T24)
                  n116 = local write "Path"(w139) -> ()
                  n117 = local write "Tab"(1) -> ()
                  n118 = call "PSTR-Update Frequency Ring.vi"("Data"=w137, "Freq Ring"=w136) -> ()  [unwired: 14 in]
                }
                frame Error {
                  n119 = call "Error Handler.vi"("error in (no error)"=w144) -> ()  [unwired: 13 in, 2 out]
                }
              }
            }
            frame True {
            }
          }
        }
        frame "next" {
          n120 = Unbundle By Name(w161) -> ("Freq"=w158:dbl[], "order"=w159:i32[], "iFreq"=w160:i32, "Run"=w148:i32)
          n121 = Increment(x=w160) -> (x+1=w151:i32)
          n122 = Index Array(array=w159, index=w151) -> (element=w147:i32)
          n123 = Index Array(array=w158, index=w147) -> (element=w156:dbl)
          n124 = call "PSTR-Progress Bar.vi"("Action"=enum16{"Init", "Seq", "Freq", "Level", "Hide"}."Freq", "Order Index"=w151, "Value Index"=w147) -> ()  [unwired: 12 in, 1 out]
          n125 = Bundle("PSTR Params"=w155, "Freq"=w156, 0, "Run"=w148) -> (w154:T34)  [unwired: 1 in]
          n126 = Bundle By Name(cluster=w161, "iFreq"=w151) -> (w153:T21)
          n127 = Enqueue Element(queue=w157, element=w154) -> ()  [unwired: 2 in, 3 out]
        }
        frame "params" {
          n128 = Unbundle By Name(w164) -> ("Stimulus"=w167:T25, "FreqSeq"=w168:T26, "LevelSeq"=w169:T27, "Seq"=w170:T28, "Response"=w171:T29, "RejThr"=w166:dbl, "Hidden.sep"=w163:dbl)
          n129 = local write "Stim"(w167) -> ()
          n130 = local write "FreqSeq"(w168) -> ()
          n131 = local write "LevelSeq"(w169) -> ()
          n132 = local write "Seq"(w170) -> ()
          n133 = local write "Response"(w171) -> ()
          n134 = local write "Separation (uV)"(w163) -> ()
          n135 = local write "RejThr"(w166) -> ()
        }
        frame "psd" {
          n136 = control-ref of="Spectrum"() -> (w175:refnum<vi>)
          n137 = call "PSTR-Replot PSDs.vi"("Data"=w174, "Graph Ref"=w175) -> ()  [unwired: 13 in, 1 out]
        }
        frame "psth" {
          n138 = control-ref of="PSTH"() -> (w183:refnum<vi>)
          n139 = call "PSTR-Show PSTHs.vi"("Data"=w182, "XYGraph"=w183, "Freq"="iFreq 2", "Separation"="Separation (uV)", "Show fits"="Show fits") -> ()  [unwired: 11 in]
        }
        frame "restore" {
          w187 = T24 {"Stimulus"={"Ear"=enum."Right", "BW (oct)"=0.3333, "Seed"=37, "Ramp (ms)"=5.0, "On time (ms)"=300.0, "Off time (ms)"=300.0, "Delay (ms)"=0.0}, "FreqSeq"={"Min (kHz)"=4.0, "Max (kHz)"=64.0, "Step (oct)"=0.5}, "LevelSeq"={"Min (dB)"=0.0, "Max (dB)"=80.0, "Step (dB)"=20.0}, "Seq"={"Order"=enum."Sequential", "Averages"=100}, "Response"={"Grass gain"=10000.0, "Window (ms)"=200.0}, "Hidden"={"Sample rate (Hz)"=100000.0, "Nfft"=2048, "save raw"=FALSE, "sep"=0.0, "Window"=enum."NONE"}, "RejThr"=15.0} ("PSTR Params")
          n140 = call "Default Config File Path.vi"() -> ("Default config file name"=w196:path)
          n141 = call "Read Anything.vi"("Type of Anything"=w187, "Section Name (Name of \"Type of Anything\")"="PSTR" ("Section Name (Name of \"Type of Anything\")"), "Path (dialog)"=w196) -> ("Error Out"=w195:errorcluster, "Found?"=w192:bool, "Anything"=w194:variant)  [unwired: 6 in]
          n142 = case shown="True" w192 {
            tunnel: w195 -> [w200 w206]
            tunnel: w194 -> [_ w205]
            tunnel: [w201 w204] -> w191
            tunnel: [w200 w203] -> w193
            tunnel: w187 -> [w201 w202]
            frame False {
            }
            frame True {
              n143 = Variant To Data(error in=w206, type=w202, Variant=w205) -> (data=w204:T24, error out=w203:errorcluster)
            }
          }
          n144 = call "Error Handler.vi"("error in (no error)"=w193) -> ()  [unwired: 13 in, 2 out]
          n145 = Build Array (concatenate)(w198, string[] ["params"]) -> (w189:string[])
        }
        frame "resume" {
          n146 = Cancel Notification(0:w213) -> ()  [unwired: 1 in, 3 out]
          n147 = control-ref of="Spectrum"() -> (w212:refnum<vi>)
          n148 = Unbundle By Name(w209) -> ("Run"=w228:i32)
          n149 = call "PSTR-Progress Bar.vi"("Data"=w209, "Action"=enum16{"Init", "Seq", "Freq", "Level", "Hide"}."Seq") -> ("error out"=w217:errorcluster)  [unwired: 13 in]
          n150 = Unbundle By Name(w209) -> ("Freq"=w226:dbl[], "order"=w227:i32[], "iFreq"=w218:i32, "iLevel"=w220:i32, "Run"=w219:i32)
          n151 = Bundle By Name(cluster=w209, "resumed"=TRUE) -> (w215:T21)
          n152 = local write "Run #"(w228) -> ()
          n153 = local write "Tab"(enum32{"Recording", "Gain", "PSTR"}."Recording" ("Tab")) -> ()
          n154 = Index Array(array=w227, index=w218) -> (element=w208:i32)
          n155 = call "PSTR-Progress Bar.vi"("Action"=enum16{"Init", "Seq", "Freq", "Level", "Hide"}."Freq", "Order Index"=w218, "Value Index"=w208, "error in (no error)"=w217) -> ("error out"=w211:errorcluster)  [unwired: 11 in]
          n156 = Index Array(array=w226, index=w208) -> (element=w225:dbl)
          n157 = call "PSTR-Restore Spont PSD.vi"("WaveformGraph in"=w212, "Data"=w209, "error in (no error)"=w211) -> ("error out"=w210:errorcluster)  [unwired: 12 in]
          n158 = Bundle("PSTR Params"=w223, "Freq"=w225, "iLevel"=w220, "Run"=w219) -> (w221:T35)  [unwired: 1 in]
          n159 = property on="Start" class="Bool"("Visible"=FALSE) -> ()  [unwired: 2 in, 2 out]
          n160 = Enqueue Element(queue=w222, element=w221, error in (no error)=w210) -> ()  [unwired: 1 in, 3 out]
        }
        frame "spont" {
          n161 = Unbundle By Name(w241) -> ("Run"=w235:i32)
          n162 = call "PSTR-Progress Bar.vi"("Action"=enum16{"Init", "Seq", "Freq", "Level", "Hide"}."Freq", "Order Index"=-1) -> ()  [unwired: 13 in, 1 out]
          n163 = Bundle("PSTR Params"=w239, nan, 0, "Run"=w235) -> (w238:cluster{"PSTR Params":T24, dbl, i32, "Run":i32})  [unwired: 1 in]
          n164 = Enqueue Element(queue=w240, element=w238) -> ()  [unwired: 2 in, 3 out]
        }
        frame "start" {
          n165 = call "PSTR-Initialize Data.vi"("PSTR Params"=w250) -> ("Data"=w246:T21, "error out"=w249:errorcluster)  [unwired: 13 in]
          n166 = case shown="No Error" w249 {
            selector: w249 -> [_ w266]
            tunnel: w248 -> [_ w267]
            tunnel: [w257 w267] -> w247
            tunnel: w246 -> [w260 _]
            tunnel: [string[] ["spont", "legend"] string[] []] -> w245
            tunnel: w244 -> [w259 w264]
            tunnel: [w258 w264] -> w243
            frame No Error {
              w251 = 0
              w252 = string[] [" "] ("Strings []")
              n167 = Unbundle By Name(w259) -> ("Run #.CAP"=w262:i16, "Experimenter"=w255:string, "Number"=w254:u32)
              n168 = call "PSTR-Progress Bar.vi"("Data"=w260, "Action"=enum16{"Init", "Seq", "Freq", "Level", "Hide"}."Seq") -> ()  [unwired: 13 in, 1 out]
              n169 = property on="iFreq" class="Ring (strict)"("Strings []"=w252, "Value"=w251) -> ()  [unwired: 2 in, 2 out]
              n170 = Increment(x=w262) -> (x+1=w256:i16)
              n171 = Bundle By Name(cluster=w259, "Run #.CAP"=w256) -> (w258:T6)
              n172 = property on="iFreq 2" class="Ring (strict)"("Strings []"=w252, "Value"=w251) -> ()  [unwired: 2 in, 2 out]
              n173 = local write "Path"(path "") -> ()
              n174 = Bundle By Name(cluster=w260, "Run"=w256, "User"=w255, "ID"=w254) -> (w257:T21)
              n175 = local write "Run #"(w256) -> ()
            }
            frame Error {
              n176 = call "Error Handler.vi"("error in (no error)"=w266) -> ()  [unwired: 13 in, 2 out]
            }
          }
        }
        frame "summary" {
          n177 = control-ref of="vsFreq"() -> (w269:refnum<vi>)
          n178 = call "PSTR-Show Summary.vi"("Data"=w268, "XYGraph"=w269) -> ()  [unwired: 14 in]
        }
      }
      n179 = Empty Array?(array=w36) -> (empty?=w44:bool)
    }
  }
  "Expt State" <- w10
  n180 = while {
    tunnel: w14 -> [w450]
    tunnel: w3 -> [w447]
    tunnel: "Expt State (in)" -> [w446]
    stop <- w449 stop-if-true
    # "MEASUREMENT THREAD"
    n181 = Dequeue Element(queue=w450) -> (element=w448:cluster{"PSTR Params":T24, dbl, i32, i32}, error out=w449:errorcluster)  [unwired: 2 in, 2 out]
    n182 = case shown="No Error" w449 {
      tunnel: w448 -> [w458 _]
      tunnel: w447 -> [w456 _]
      tunnel: w446 -> [w455 _]
      frame No Error {
        n183 = Unbundle(w458) -> ("PSTR Params"=w457:T24, w454:dbl, w452:i32, w451:i32)
        n184 = while {
          tunnel: w457 -> [w471]
          tunnel: w456 -> [w470]
          tunnel: w455 -> [w469]
          tunnel: w454 -> [w468]
          shift-right: [w467] -> _
          shift-left: _ -> [w466]
          shift-right: [w464] -> _
          shift-left: PSTR-Measurement_State."Init" ("Enum") -> [w465]
          shift-right: [w463] -> _
          shift-left: _ -> [w462]
          tunnel: w452 -> [w460]
          tunnel: w451 -> [w459]
          stop <- w461 stop-if-true
          n185 = case shown="\"Init\", Default" w465 {
            tunnel: w471 -> [w479 w507 _ _]
            tunnel: w470 -> [_ _ w537 _]
            tunnel: w469 -> [w473 w504 _ _]
            tunnel: w468 -> [w485 w501 _ _]
            tunnel: [w483 w515 w534 w575] -> w467
            tunnel: w466 -> [_ w489 w542 w575]
            tunnel: [w484 w494 PSTR-Measurement_State."End" ("f") PSTR-Measurement_State."Next" ("f")] -> w464
            tunnel: [w478 w495 w538 w580] -> w463
            tunnel: w462 -> [_ w499 _ w580]
            tunnel: [_ _ _ w582] -> w461
            tunnel: w460 -> [w475 _ _ _]
            tunnel: w459 -> [_ w505 _ _]
            frame "Init", Default {
              n186 = Unbundle By Name(w473) -> ("Data Folder"=w472:path)
              n187 = call "PSTR-Initialize.vi"("PSTR Params"=w479, "Data folder"=w472, "Freq (kHz)"=w485) -> ("Runtime"=w482:T38, "error out"=w481:errorcluster)  [unwired: 11 in]
              n188 = Decrement(x=w475) -> (x-1=w474:i32)
              n189 = call "PSTR-Initialize Analysis.vi"("Runtime in"=w482, "PSTR Params"=w479, "error in (no error)"=w481) -> ("Runtime out"=w480:T38, "error out"=w478:errorcluster)  [unwired: 11 in]
              n190 = Bundle By Name(cluster=w480, "iLevel"=w474) -> (w483:T38)
              n191 = Select(t=PSTR-Measurement_State."End" ("Enum"), s=w478, f=PSTR-Measurement_State."Next") -> (s? t:f=w484:T36)
            }
            frame "Next" {
              w514 = 0 ("nacc")
              n192 = Unbundle By Name(w504) -> ("Data Folder"=w500:path, "Experimenter"=w503:string, "Number"=w502:u32)
              n193 = Unbundle By Name(w507) -> ("Hidden.save raw"=w506:bool)
              n194 = Unbundle By Name(w489) -> ("iLevel"=w516:i32, "spont"=w493:bool)
              n195 = Unbundle By Name(w489) -> ("trialLen"=w487:i32)
              n196 = Unbundle By Name(w489) -> ("Nfft"=w513:i32)
              n197 = Increment(x=w516) -> (x+1=w490:i32)
              n198 = case shown="True" w506 {
                tunnel: w505 -> [_ w529]
                tunnel: w503 -> [_ w531]
                tunnel: w502 -> [_ w530]
                tunnel: w501 -> [_ w528]
                tunnel: w490 -> [_ w527]
                tunnel: w500 -> [_ w526]
                tunnel: [w518 w521] -> w495
                tunnel: [_ w520] -> w498
                tunnel: w499 -> [w518 w519]
                frame False {
                }
                frame True {
                  n199 = Format Into String(format string="%s%d-%d-PSTR.%#_4gkHz.%d.f64", w531, w530, w529, w528, w527) -> (resulting string=w525:string)  [unwired: 2 in, 1 out]
                  n200 = Build Path(base path=w526, name or relative path=w525) -> (appended path=w524:path)
                  n201 = Open/Create/Replace File(file path (use dialog)=w524, error in=w519, operation (0:open)=T37."create", access (0:read/write)=enum16{"read/write", "read-only", "write-only"}."write-only") -> (refnum out=w520:refnum<file>, error out=w521:errorcluster)  [unwired: 2 in, 1 out]
                }
              }
              n202 = Select(t=-1, s=w493, f=w490) -> (s? t:f=w491:i32)
              n203 = Quotient & Remainder(x=w513, y=2) -> (floor(x/y)=w511:i32)  [unwired: 1 out]
              n204 = Increment(x=w511) -> (x+1=w510:i32)
              n205 = call "PSTR-Progress Bar.vi"("Action"=enum16{"Init", "Seq", "Freq", "Level", "Hide"}."Level", "Order Index"=w491) -> ()  [unwired: 13 in, 1 out]
              n206 = Initialize Array(0.0 ("element"), w487) -> (w486:dbl[])
              n207 = Initialize Array(0.0, w510) -> (w508:dbl[])
              n208 = Bundle By Name(cluster=w489, "iLevel"=w490, "nacc"=w514, "nrej"=w514, "Neural"=w508, "Micro"=w508, "PSTR"=w486, "raw"=w498) -> (w515:T38)
              n209 = Select(t=PSTR-Measurement_State."End" ("Enum"), s=w495, f=PSTR-Measurement_State."Measure") -> (s? t:f=w494:T36)
            }
            frame "Measure" {
              n210 = while {
                shift-right: [w545] -> w539
                shift-left: w542 -> [w562]
                tunnel: [w548] -> w540
                tunnel: w537 -> [w555]
                tunnel: [w552] -> w536
                tunnel: [w551] -> w533
                stop <- w556 stop-if-true
                n211 = call "Data Available Queue.vi"() -> ("AI Waveforms"=w564:dbl[][], "error out"=w563:errorcluster)  [unwired: 11 in, 3 out]
                n212 = Index Array(array=w564) -> (element=w559:dbl[])  [unwired: 2 in]
                n213 = Wait on Notification(notifier=w555, timeout in ms (-1)=0) -> (notifier out=w552:refnum<notifier>, notification=w551:bool)  [unwired: 2 in, 2 out]
                n214 = control-ref of="Spectrum"() -> (w547:refnum<vi>)
                n215 = call "PSTR-Process Frame.vi"("Runtime in"=w562, "Override"="Override", "RejThr"="RejThr", "data"=w559, "error in (no error)"=w563) -> ("Runtime out"=w546:T38, "reject"=→"reject":bool, "done"=w558:bool, "waveform"=→"Waveform":cluster{dbl, "dx":dbl, "Y":dbl[]}[], "status"=→"Status":string, "error out"=w549:errorcluster)  [unwired: 5 in]
                n216 = call "PSTR-Plot PSDs.vi"("Runtime in"=w546, "Graph"=w547, "error in (no error)"=w549) -> ("Runtime out"=w545:T38, "error out"=w548:errorcluster)  [unwired: 11 in]
                n217 = Or(x=w558, y=w551) -> (x .or. y?=w556:bool)
                n218 = Wait (ms)(milliseconds to wait=u32 10) -> ()  [unwired: 1 out]
              }
              n219 = call "PSTR-AO Thread.vi"("Runtime"=w542, "abort"=w537) -> ("error out"=w541:errorcluster)  [unwired: 13 in]
              n220 = Bundle By Name(cluster=w539, "abort"=w533) -> (w534:T38)
              n221 = Send Notification(notification=FALSE, notifier=w536) -> ()  [unwired: 1 in, 2 out]
              n222 = Merge Errors(w541, w540) -> (w538:errorcluster)
            }
            frame "End" {
              n223 = Unbundle By Name(w575) -> ("spont"=w570:bool, "iLevel"=w576:i32, "Level"=w585:dbl[])
              n224 = Unbundle By Name(w575) -> ("raw"=w577:refnum<file>)
              n225 = Unbundle By Name(w575) -> ("Neural"=w574:dbl[], "Micro"=w573:dbl[], "PSTR"=w567:dbl[], "nacc"=w566:i32)
              n226 = Unbundle By Name(w575) -> ("abort"=w579:bool)
              n227 = Array Size(array=w585) -> (size(s)=w584:i32)
              n228 = Not A Number/Path/Refnum?(number/path/refnum=w577) -> (NaN/Path/Refnum?=w578:bool)
              n229 = Build Array(w574, w573) -> (w572:dbl[][])
              n230 = Decrement(x=w584) -> (x-1=w583:i32)
              n231 = case shown="False" w578 {
                tunnel: w577 -> [w587 _]
                frame False {
                  n232 = Close File(refnum=w587) -> ()  [unwired: 1 in, 2 out]
                }
                frame True {
                }
              }
              n233 = Divide(x=w572, y=w566) -> (x/y=w571:dbl[][])
              n234 = Divide(x=w567, y=w566) -> (x/y=w565:dbl[])
              n235 = Equal?(x=w576, y=w583) -> (x = y?=w581:bool)
              n236 = Compound Arithmetic op=OR(w581, w579, w580) -> (w582:bool)
              n237 = Bundle By Name(cluster=T7 {"iLevel"=0, "done"=FALSE, "abort"=FALSE, "PSD"=[], "error"={"status"=FALSE, "code"=0, "source"=""}, "spont"=FALSE, "PSTH"=[]} ("Value (Signaling)"), "spont"=w570, "iLevel"=w576, "done"=w581, "abort"=w579, "PSD"=w571, "PSTH"=w565, "error"=w580) -> (w568:T7)
              n238 = property on="Result" class="Clust (strict)"("Val(Sgnl)"=w568) -> ()  [unwired: 2 in, 2 out]
            }
          }
        }
      }
      frame Error {
      }
    }
  }
